vi "CheckNTDataStart.vi"(11 "ValToCheck":dbl) -> (3 "GetData":bool)   [LabVIEW 2018]
uses:
  Swerve/SwerveGlobals.vi
  <vilib>/Rock Robotics/Network Tables/NT Write Boolean.vi
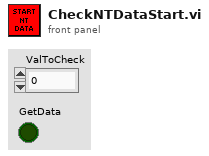
[diagram p1: front panel]
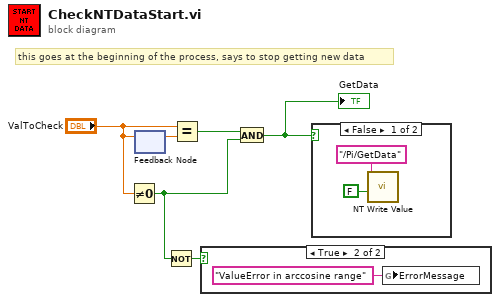
[diagram p0: block diagram]
diagram:
  # "this goes at the beginning of the process, says to stop getting new data"
  n1 = Not Equal To 0?(x="ValToCheck") -> (x != 0?=w2:bool)
  n2 = feedback #1() -> (w5:dbl)  [unwired: 1 in]
  n3 = feedback-in #1("ValToCheck") -> ()
  n4 = Not(x=w2) -> (.not. x?=w3:bool)
  n5 = Equal?(x="ValToCheck", y=w5) -> (x = y?=w4:bool)
  n6 = case shown="True" w3 {
    frame False {
    }
    frame True {
      n7 = global write "SwerveGlobals.vi" "ErrorMessage"("ValueError in arccosine range" ("ErrorMessage")) -> ()
    }
  }
  n8 = And(x=w4, y=w2) -> (x .and. y?=w1:bool)
  "GetData" <- w1
  n9 = case shown="False" w1 {
    frame False {
      n10 = call-poly <vilib>:"NT Write Value.vi"("Boolean"=FALSE, "Name"="/Pi/GetData" ("Client Name")) -> ()  [unwired: 9 in, 1 out]
    }
    frame True {
    }
  }
